vi "Self Queue.vi"(9 "Priority?":bool, 10 "Msg Strategy":refnum<class "Msg Strategy.lvclass">, 11 "Queue in":refnum<class "Queue.lvclass">) -> (3 "Queue out":refnum<class "Queue.lvclass">)   [LabVIEW 2021, in "jettl.lvlib" / "Queue.lvclass"]
uses:
  Queue.lvclass
  Msg Strategy/Msg Strategy.lvclass
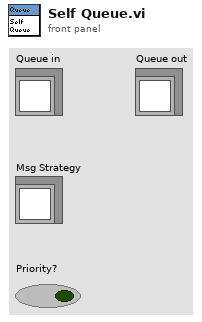
[diagram p1: front panel]
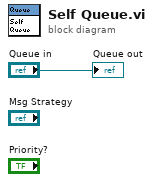
[diagram p0: block diagram]
diagram:
  "Queue out" <- "Queue in"
